vi "nivelMaxRef.vi"(8 "error in (no error)":errorcluster, 9 "Tm":dbl=60.0, 10 "N":dbl=1.0, 11 "Prueba08 in":refnum<class "Prueba03.lvclass">) -> (0 "error out":errorcluster, 2 "ms":string[](array[string]), 3 "Prueba08 out":refnum<class "Prueba03.lvclass">, 4 "nivelMaxRef":dbl, 5 "tablaNivelMaxRef":string[](array[string]), 6 "tablaTipoPondTemp":string[](array[string]))   [LabVIEW 2019]
uses:
  Prueba/Prueba.lvclass
  Prueba03.lvclass
  D:/REPO/GitHub/procal/Pruebas/Prueba/Prueba.lvclass
panel:
  out "Tabla":dbl[](array[numeric]) format="%#.1f"
  out "Leq":dbl[](array[numeric])
  out "nivelMaxRef":string
  out "LA":dbl
  out "tipoPondTemp":string
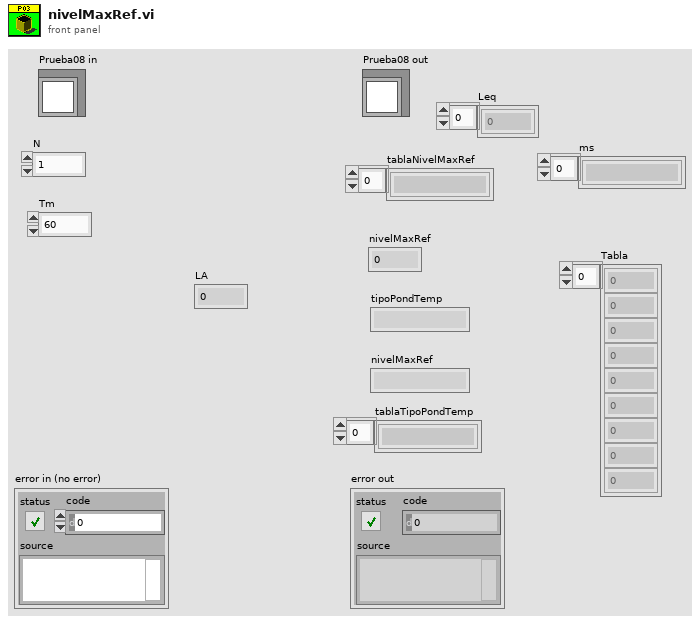
[diagram p1: front panel]
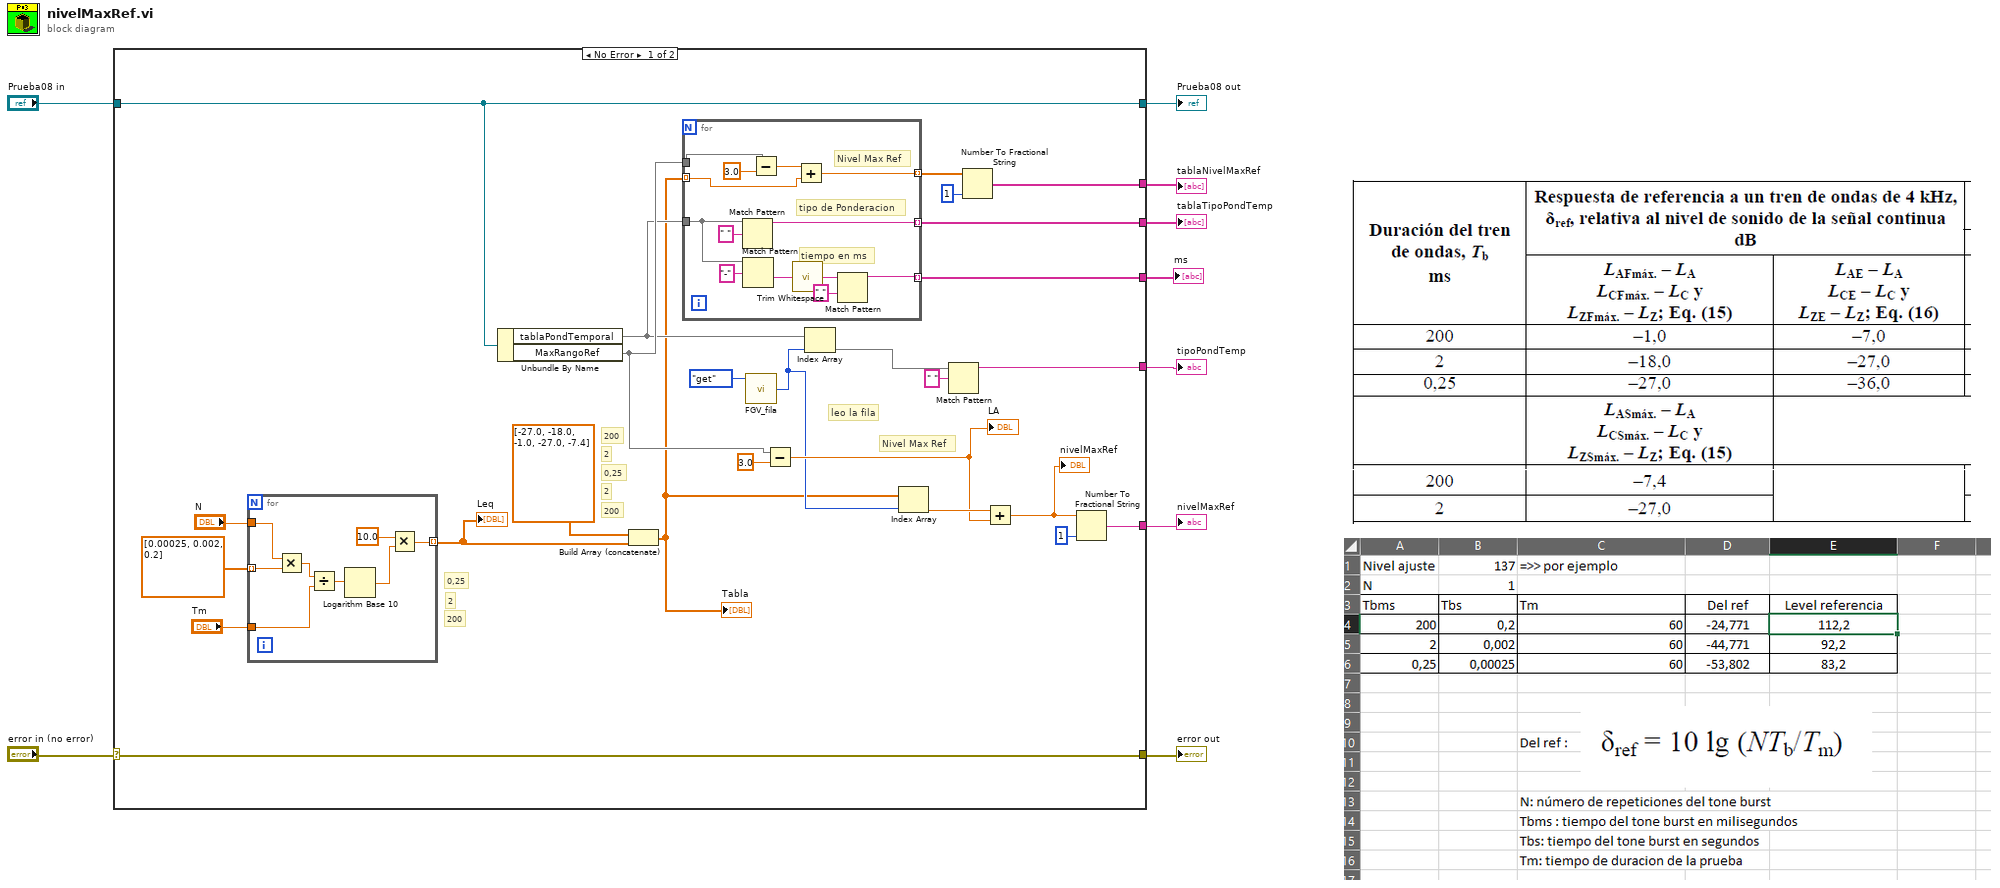
[diagram p0: block diagram]
diagram:
  n1 = case shown="No Error" "error in (no error)" {
    selector: "error in (no error)" -> [w30 w58]
    tunnel: "Prueba08 in" -> [w29 w57]
    tunnel: [w34 _] -> w8
    tunnel: [w30 w58] -> w6
    tunnel: [w29 w57] -> w5
    tunnel: [w24 _] -> w4
    tunnel: [w20 _] -> w3
    tunnel: [w18 _] -> w2
    tunnel: [w17 _] -> w1
    frame No Error {
      # "2"
      # "200"
      # "0,25"
      # "200"
      # "2"
      # "0,25"
      # "2"
      # "200"
      # "Nivel Max Ref"
      # "leo la fila"
      n2 = for {
        tunnel: dbl[] [0.00025, 0.002, 0.2] -> [w39] mode=indexing
        tunnel: [w38] -> w11 mode=indexing
        tunnel: "N" -> [w37]
        tunnel: "Tm" -> [w36]
        n3 = Multiply(x=w37, y=w39) -> (x*y=w43:dbl)
        n4 = Divide(x=w43, y=w36) -> (x/y=w42:dbl)
        n5 = Logarithm Base 10(1:w42) -> (0:w41:dbl)
        n6 = Multiply(x=10.0, y=w41) -> (x*y=w38:dbl)
      }
      "Leq" <- w11
      n7 = Unbundle By Name(w29) -> ("tablaPondTemporal"=w19, "MaxRangoRef"=w23)
      n8 = Build Array (concatenate)(dbl[] [-27.0, -18.0, -1.0, -27.0, -7.4], w11) -> (w10:dbl[])
      "Tabla" <- w10
      n9 = for {
        tunnel: w23 -> [w55]
        tunnel: w10 -> [w53] mode=indexing
        tunnel: [w52] -> w22 mode=indexing
        tunnel: w19 -> [w49]
        tunnel: [w50] -> w18 mode=indexing
        tunnel: [w44] -> w17 mode=indexing
        # "Nivel Max Ref"
        # "tiempo en ms"
        # "tipo de Ponderacion"
        n10 = Match Pattern(string=w49, regular expression=" ") -> (before substring=w50:string)  [unwired: 1 in, 3 out]
        n11 = Match Pattern(string=w49, regular expression="-") -> (after substring=w47:string)  [unwired: 1 in, 3 out]
        n12 = Subtract(x=w55, y=3.0) -> (x-y=w54:dbl)
        n13 = call <vilib>:"Trim Whitespace.vi"("string"=w47) -> ("trimmed string"=w46:string)  [unwired: 1 in]
        n14 = Add(x=w54, y=w53) -> (x+y=w52:dbl)
        n15 = Match Pattern(string=w46, regular expression=" ") -> (before substring=w44:string)  [unwired: 1 in, 3 out]
      }
      n16 = call "FGV_fila.vi"("action"=enum16{"increment", "set_start", "get"}."get") -> ("fila out"=w16:i32)  [unwired: 3 in, 1 out]
      n17 = Subtract(x=w23, y=3.0) -> (x-y=w27:dbl)
      "LA" <- w27
      n18 = Index Array(array=w19, index=w16) -> (element=w28)
      n19 = Index Array(array=w10, index=w16) -> (element=w31:dbl)
      n20 = Match Pattern(string=w28, regular expression=" ") -> (before substring=w34:string)  [unwired: 1 in, 3 out]
      n21 = Number To Fractional String(number=w22, precision (6)=i16 1) -> (F-format string=w20:string[])  [unwired: 2 in]
      n22 = Add(x=w31, y=w27) -> (x+y=w26:dbl)
      "nivelMaxRef" <- w26
      n23 = Number To Fractional String(number=w26, precision (6)=i16 1) -> (F-format string=w24:string)  [unwired: 2 in]
    }
    frame Error {
    }
  }
  "Prueba08 out" <- w5
  "error out" <- w6
  "tipoPondTemp" <- w8
  "nivelMaxRef" <- w4
  "tablaNivelMaxRef" <- w3
  "tablaTipoPondTemp" <- w2
  "ms" <- w1
